vi "Query DisLevel.vi"(8 "error in (no error)":errorcluster, 11 "CS++MCS in":refnum<class "CS++MCS.lvclass">) -> (0 "error out":errorcluster, 2 "Discriminator Level":dbl[unit], 3 "CS++MCS out":refnum<class "CS++MCS.lvclass">)   [LabVIEW 2016, in "CS++MCS.lvlib" / "CS++MCS.lvclass"]
doc: "This VI reads out the Discriminator Level from the device."
uses:
  CS++MCS.lvclass
  CSPP_Core/Classes/CS++ProcessVariables/ProcessVariable/PV.lvclass
  PV-Enum.ctl
  CSPP_Core/Classes/CS++ProcessVariables/ProcessVariable/PV.lvclass/PV.ctl
  CS++MCS.lvclass/CS++MCS.ctl
  CSPP_Core/Classes/CS++ProcessVariables/ProcessVariable/Write Data.vi
  CSPP_Core/Classes/CS++ProcessVariables/ProcessVariable/Write Timestamp.vi
  CSPP_Core/Classes/CS++ProcessVariables/ProcessVariable/Write Quality.vi
  CSPP_Core/Classes/CS++ProcessVariables/ProcessVariable/Write status.vi
  CSPP_Core/Classes/CS++ProcessVariables/PVConnection/PVConnection.lvclass
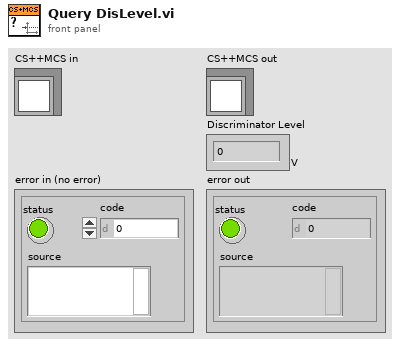
[diagram p1: front panel]
types:
  T1 = typedef "CS++MCS.lvlib/CS++MCS.lvclass/PV-Enum.ctl" = enum16{"Counts/I32", "TotalCounts/I32", "Status/I8", "BinWidth/Dbl", "NofBins/I32", "NofRecords /I32", "DiscLvl/Dbl", "TrigLvl/Dbl", "DiscSlope/U16", "TrigSlope/U16", "ActWaveform/AWfm|0:1"}
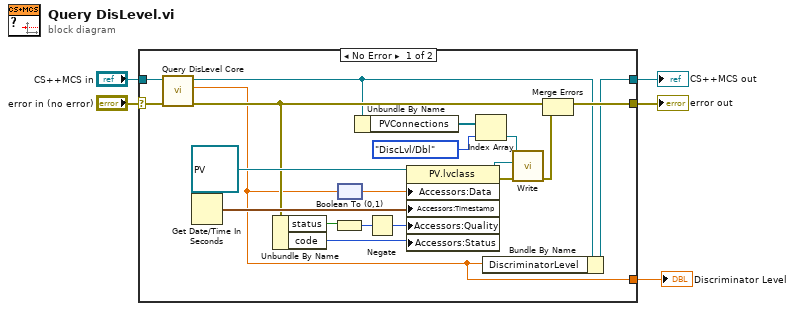
[diagram p0: block diagram]
diagram:
  n1 = case shown="No Error" "error in (no error)" {
    selector: "error in (no error)" -> [w24 w27]
    tunnel: [w9 w27] -> w4
    tunnel: [w8 w26] -> w2
    tunnel: "CS++MCS in" -> [w25 w26]
    tunnel: [w6 _] -> w1
    frame No Error {
      n2 = call-dynamic "Query DisLevel Core.vi"("error in (no error)"=w24, "CS++MCS in"=w25) -> ("error out"=w10:errorcluster, "Discriminator Level"=w6:dbl[unit], "CS++MCS out"=w7:refnum<class "CS++MCS.lvclass">)  [unwired: 7 in]
      n3 = Get Date/Time In Seconds() -> (seconds since 1Jan1904=w15:timestamp)
      n4 = Unbundle By Name(w10) -> ("status"=w19:bool, "code"=w21:i32)
      n5 = Boolean To (0,1)(Boolean=w19) -> (0, 1=w20:i16)
      n6 = node(w6) -> (w12:dbl)
      n7 = Unbundle By Name(w7) -> ("PVConnections"=w23:refnum<class "PVConnection.lvclass">[])
      n8 = Negate(x=w20) -> (-x=w22:i16)
      n9 = property class="PV.lvclass"(reference=refnum<class "PV.lvclass"> refnum ("PV"), "Accessors:Data"=w12, "Accessors:Timestamp"=w15, "Accessors:Quality"=w22, "Accessors:Status"=w21) -> (reference out=w18:refnum<class "PV.lvclass">, error out=w17:errorcluster)  [unwired: 1 in]
      n10 = Index Array(array=w23, index=PV-Enum."DiscLvl/Dbl" ("PV-Enum")) -> (element=w14:refnum<class "PVConnection.lvclass">)
      n11 = Bundle By Name(cluster=w7, "DiscriminatorLevel"=w6) -> (w8:refnum<class "CS++MCS.lvclass">)
      n12 = call "Write.vi"("error in (no error)"=w17, "PV"=w18, "PVConnection in"=w14) -> ("error out"=w13:errorcluster)  [unwired: 7 in, 1 out]
      n13 = Merge Errors(w10, w13) -> (w9:errorcluster)
    }
    frame Error {
    }
  }
  "error out" <- w4
  "CS++MCS out" <- w2
  "Discriminator Level" <- w1
